vi "状态告警区.vi"(11 "数组":u16[](array[numeric]) format="%04xH") -> (3 "状态告警区":T1 {"工作状态" items=["空闲"=0, "水样测试"=1, "标样核查"=2, "零点核查"=3, "跨度核查"=4, "空白测试"=5, "平行样测试"=6, "加标回收"=7, "空白校准"=8, "标样校准"=9, "初始化（清洗）"=10, "调试"=22, "填充管路"=30, "清洗管路"=31, "清洗反应杯"=32]; "告警代码" items=["无告警", "缺试剂告警", "缺水样告警", "缺蒸馏水告警", "缺标液告警", "仪表漏液告警", "标定异常告警", "超量程告警", "加热异常", "低试剂预警", "超上限告警", "超下限告警", "仪表内部其他异常", "滴定异常告警", "电极异常告警", "量程切换告警", "参数设置告警", "PH电极电位异常", "电导率电极异常", "浊度光度异常", "溶解氧电极异常", "溶解氧光强异常", "温度异常告警", "PH异常告警", "溶解氧异常告警", "电导率异常告警", "浊度异常告警", "叶绿素异常告警", "藻密度异常告警", "蓝绿藻异常告警", "ORP异常告警", "氨氮异常告警", "清洁刷异常告警", "SD卡异常告警", "蓝牙异常告警", "Wifi异常告警", "流程异常告警"]; "故障代码" items=["无故障", "电机故障", "温度故障", "通讯故障", "滴定故障"]})   [LabVIEW 2016, in "斯坦道CODMn新电路板.lvlib"]
panel:
  # "共占用29 WORD"
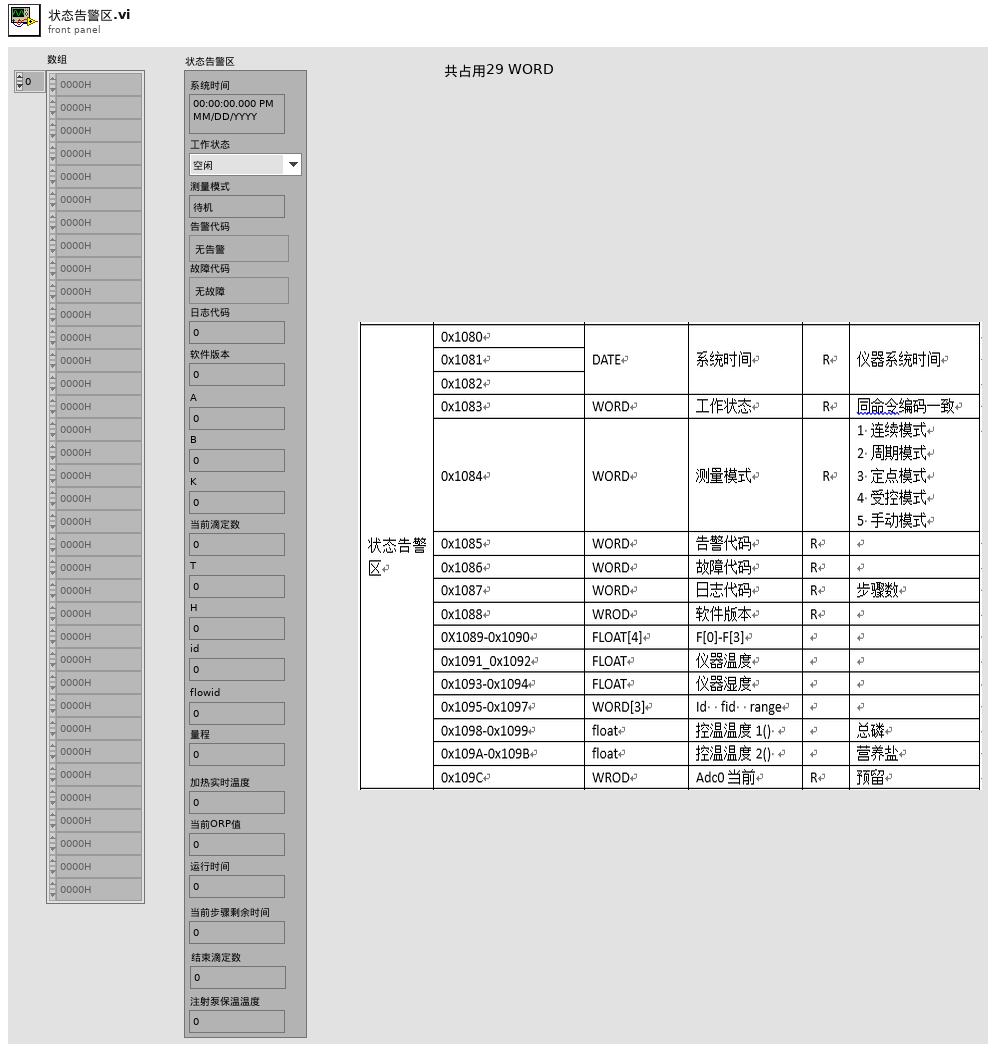
[diagram p1: front panel]
types:
  T1 = cluster{"系统时间":timestamp, "工作状态":u16, "测量模式":enum16{"待机", "连续模式", "周期模式", "定点模式", "受控模式", "手动模式"}, "告警代码":u16, "故障代码":u16, "日志代码":u16, "软件版本":u16, "A":sgl, "B":sgl, "K":sgl, "当前滴定数":sgl, "T":sgl, "H":sgl, "id":u16, "flowid":u16, "量程":u16, "加热实时温度":sgl, "当前ORP值":sgl, "运行时间":sgl, "当前步骤剩余时间":sgl, "结束滴定数":sgl, "注射泵保温温度":sgl}
  T2 = cluster{"系统时间":timestamp, "工作状态":enum16{"空闲", "水样测试", "标样核查", "零点核查", "跨度核查", "空白测试", "平行样测试", "加标回收", "空白校准", "标样校准", "初始化（清洗）"}, "测量模式":enum16{"待机", "连续模式", "周期模式", "定点模式", "受控模式", "手动模式"}, "告警代码":u16, "故障代码":u16, "日志代码":u16, "软件版本":u16, "A":sgl, "B":sgl, "K":sgl, "当前滴定数":sgl, "T":sgl, "H":sgl, "id":u16, "flowid":u16, "量程":u16, "加热实时温度":sgl, "当前ORP值":sgl, "运行时间":sgl, "当前步骤剩余时间":sgl, "结束滴定数":sgl, "注射泵保温温度":sgl}
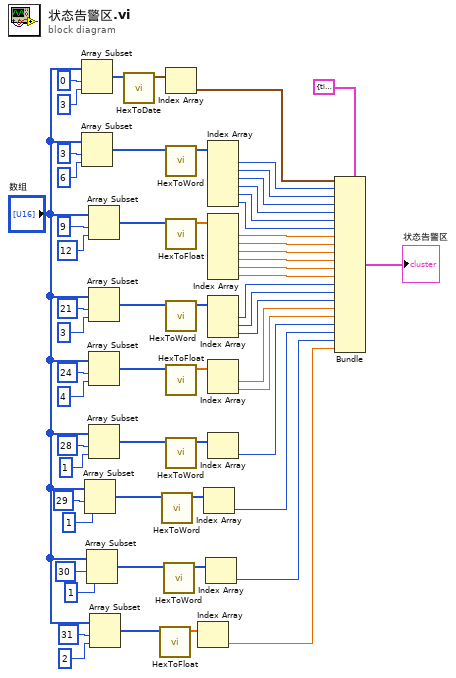
[diagram p0: block diagram]
diagram:
  n1 = Array Subset(array="数组", index=0 ("索引"), length=3 ("长度")) -> (w59:u16[])
  n2 = Array Subset(array="数组", index=3 ("索引"), length=6 ("长度")) -> (w54:u16[])
  n3 = Array Subset(array="数组", index=29 ("索引"), length=1 ("长度")) -> (w18:u16[])
  n4 = Array Subset(array="数组", index=30 ("索引"), length=1 ("长度")) -> (w11:u16[])
  n5 = Array Subset(array="数组", index=9 ("索引"), length=12 ("长度")) -> (w44:u16[])
  n6 = Array Subset(array="数组", index=21 ("索引"), length=3 ("索引")) -> (w34:u16[])
  n7 = Array Subset(array="数组", index=24 ("索引"), length=4 ("索引")) -> (w27:u16[])
  n8 = Array Subset(array="数组", index=28 ("索引"), length=1 ("长度")) -> (w22:u16[])
  n9 = Array Subset(array="数组", index=31 ("索引"), length=2 ("索引")) -> (w6:u16[])
  n10 = call "HexToDate.vi"("数组"=w59) -> ("DATE"=w56:timestamp[])  [unwired: 10 in]
  n11 = call "HexToFloat.vi"("数组"=w6) -> ("FLOAT"=w5:sgl[])  [unwired: 10 in]
  n12 = call "HexToWord.vi"("数组"=w18) -> ("WORD"=w17:u16[])  [unwired: 10 in]
  n13 = call "HexToWord.vi"("数组"=w11) -> ("WORD"=w12:u16[])  [unwired: 10 in]
  n14 = Index Array(array=w56) -> (element=w55:timestamp)  [unwired: 1 in]
  n15 = call "HexToWord.vi"("数组"=w54) -> ("WORD"=w53:u16[])  [unwired: 10 in]
  n16 = call "HexToFloat.vi"("数组"=w44) -> ("FLOAT"=w43:sgl[])  [unwired: 10 in]
  n17 = call "HexToWord.vi"("数组"=w34) -> ("WORD"=w33:u16[])  [unwired: 10 in]
  n18 = call "HexToFloat.vi"("数组"=w27) -> ("FLOAT"=w26:sgl[])  [unwired: 10 in]
  n19 = call "HexToWord.vi"("数组"=w22) -> ("WORD"=w23:u16[])  [unwired: 10 in]
  n20 = Index Array(array=w5) -> (element=w1:sgl)  [unwired: 1 in]
  n21 = Index Array(array=w17) -> (element=w16:u16)  [unwired: 1 in]
  n22 = Index Array(array=w12) -> (element=w9:u16)  [unwired: 1 in]
  n23 = Index Array(array=w53) -> (element #1=w52:u16, element #2=w51:u16, element #3=w50:u16, element #4=w49:u16, element #5=w48:u16, element #6=w47:u16)  [unwired: 6 in]
  n24 = Index Array(array=w43) -> (element #1=w42:sgl, element #2=w41:sgl, element #3=w40:sgl, element #4=w39:sgl, element #5=w38:sgl, element #6=w37:sgl)  [unwired: 6 in]
  n25 = Index Array(array=w33) -> (element #1=w32:u16, element #2=w31:u16, element #3=w30:u16)  [unwired: 3 in]
  n26 = Index Array(array=w26) -> (element #1=w25:sgl, element #2=w24:sgl)  [unwired: 2 in]
  n27 = Index Array(array=w23) -> (element=w20:u16)  [unwired: 1 in]
  n28 = Bundle(cluster=T2 {"系统时间"=timestamp(0 s since 1904-01-01), "工作状态"=enum."空闲", "测量模式"=enum."待机", "告警代码"=0, "故障代码"=0, "日志代码"=0, "软件版本"=0, "A"=0.0, "B"=0.0, "K"=0.0, "当前滴定数"=0.0, "T"=0.0, "H"=0.0, "id"=0, "flowid"=0, "量程"=0, "加热实时温度"=0.0, "当前ORP值"=0.0, "运行时间"=0.0, "当前步骤剩余时间"=0.0, "结束滴定数"=0.0, "注射泵保温温度"=0.0} ("状态告警区"), "系统时间"=w55, "工作状态"=w52, "测量模式"=w51, "告警代码"=w50, "故障代码"=w49, "日志代码"=w48, "软件版本"=w47, "A"=w42, "B"=w41, "K"=w40, "当前滴定数"=w39, "T"=w38, "H"=w37, "id"=w32, "flowid"=w31, "量程"=w30, "加热实时温度"=w25, "当前ORP值"=w24, "运行时间"=w20, "当前步骤剩余时间"=w16, "结束滴定数"=w9, "注射泵保温温度"=w1) -> (→"状态告警区":T2)
